vi "Create File.vi"(11 "path":path) -> (0 "error out":errorcluster, 3 "path out":path)   [LabVIEW 2013]
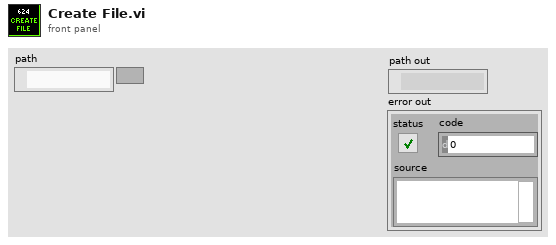
[diagram p1: front panel]
types:
  T1 = enum16{"open", "replace", "create", "open or create", "replace or create", "replace or create with confirmation"}
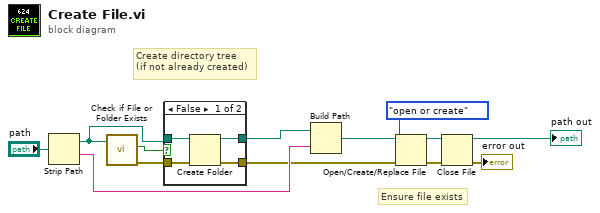
[diagram p0: block diagram]
diagram:
  # "Ensure file exists"
  # "Create directory tree\n(if not already created)"
  n1 = Strip Path(path="path") -> (stripped path=w1:path, name=w9:string)
  n2 = call <vilib>:"Check if File or Folder Exists.vi"("path"=w1) -> ("error out"=w11:errorcluster, "file or folder exists?"=w12:bool)  [unwired: 8 in, 1 out]
  n3 = case shown="False" w12 {
    tunnel: w1 -> [w17 w18]
    tunnel: w11 -> [w16 w19]
    tunnel: [w15 w18] -> w10
    tunnel: [w14 w19] -> w4
    frame False {
      n4 = Create Folder(path (use dialog)=w17, error in=w16) -> (created path=w15:path, error out=w14:errorcluster)  [unwired: 1 in, 1 out]
    }
    frame True {
    }
  }
  n5 = Build Path(base path=w10, name or relative path=w9) -> (appended path=w7:path)
  n6 = Open/Create/Replace File(file path (use dialog)=w7, error in=w4, operation (0:open)=T1."open or create") -> (refnum out=w5:refnum<file>, error out=w6:errorcluster)  [unwired: 3 in, 1 out]
  n7 = Close File(refnum=w5, error in=w6) -> (path=→"path out":path, error out=→"error out":errorcluster)
